vi "_emi_Version to VI tags.vi"(0 "vi Refnum in":refnum<vi>, 7 "Version Info":T1={"Name"="Default Name", "Major"=0, "Minor"=0, "Fix"=0, "Build"=0, "Type"=enum."Alfa", "Dev"=FALSE, "Version Name"="", "Date"=timestamp(0 s since 1904-01-01)} {"Date" format="%<%y%m%d>T"}, 11 "error in":errorcluster) -> (4 "vi Refnum out":refnum<vi>, 15 "error out":errorcluster)   [LabVIEW 2010]
doc: "Writes teh *Version info Cluster top the VI tags and History revision.\n\nOn error, no error signal is transmitted on. Performes even on error in"
uses:
  emi_Version Info.ctl
  <vilib>/UserTags/UserTags.lvlib
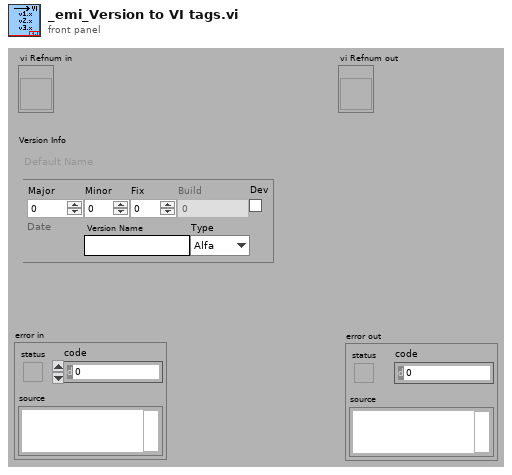
[diagram p1: front panel]
types:
  T1 = typedef "emi_Version Info.ctl" = cluster{"Name":string, "Major":i16, "Minor":i16, "Fix":i16, "Build":i32, "Type":enum16{"Alfa", "Beta", "Stable"}, "Dev":bool, "Version Name":string, "Date":timestamp}
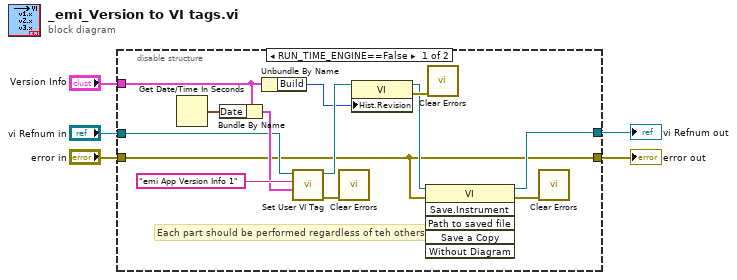
[diagram p0: block diagram]
diagram:
  n1 = disable-structure shown="RUN_TIME_ENGINE==False" {
    disable-tunnel: "vi Refnum in" -> [w15 w20]
    disable-tunnel: "Version Info" -> [w13 _]
    disable-tunnel: [w10 w20] -> w3
    disable-tunnel: "error in" -> [w6 w19]
    disable-tunnel: [w6 w19] -> w1
    frame condition #0 (active) {
      # "Each part should be performed regardless of teh others"
      n2 = Get Date/Time In Seconds() -> (seconds since 1Jan1904=w17:timestamp)
      n3 = Bundle By Name(cluster=w13, "Date"=w17) -> (w16:T1)
      n4 = Unbundle By Name(w13) -> ("Build"=w12:i32)
      n5 = call <vilib>:"Set User VI Tag.vi"("Value"=w16, "Tag Name"="emi App Version Info 1", "VI Refnum"=w15) -> ("error out"=w7:errorcluster, "dup VI Refnum"=w14:refnum<vi>)  [unwired: 6 in, 1 out]
      n6 = call <vilib>:"Clear Errors.vi"("error in (no error)"=w7) -> ()  [unwired: 6 in, 1 out]
      n7 = property class="VI"(reference=w14, "Hist.Revision"=w12) -> (reference out=w9:refnum<vi>, error out=w11:errorcluster)  [unwired: 1 in]
      n8 = invoke class="VI" method="Save.Instrument"(reference=w9, error in=w6) -> (reference out=w10:refnum<vi>, error out=w8:errorcluster)  [unwired: 4 in, 4 out]
      n9 = call <vilib>:"Clear Errors.vi"("error in (no error)"=w11) -> ()  [unwired: 6 in, 1 out]
      n10 = call <vilib>:"Clear Errors.vi"("error in (no error)"=w8) -> ()  [unwired: 6 in, 1 out]
    }
    frame condition #1 {
    }
  }
  "error out" <- w1
  "vi Refnum out" <- w3
